vi "Write BBM Slot.vi"(0 "WorkTable Class in":refnum<class "WorkTable Class.lvclass">, 5 "Chuck Number":u32, 7 "Slot Number":u32, 9 "new element/subarray":T1, 11 "error in (no error)":errorcluster) -> (4 "WorkTable Class out":refnum<class "WorkTable Class.lvclass">, 15 "error out":errorcluster)   [LabVIEW 2011, in "WorkTable Class.lvclass"]
uses:
  WorkTable Class.lvclass
  Vec3d Class/Vec3d Class.lvclass
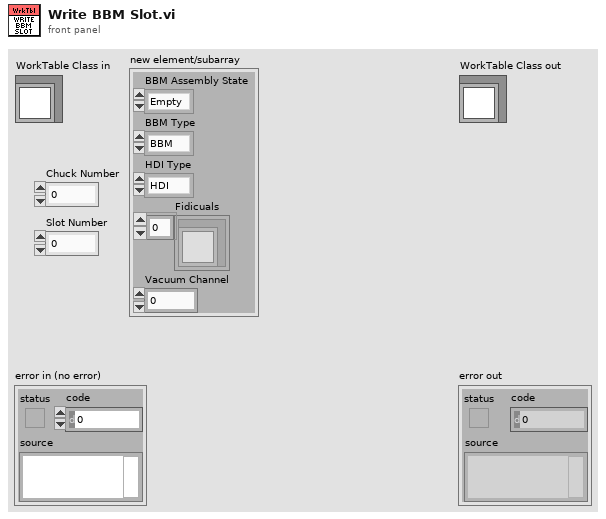
[diagram p1: front panel]
types:
  T1 = cluster{"BBM Assembly State":enum16{"Empty", "Unglued", "Stamped", "PartOnTop", "Weighted"}, "BBM Type":enum16{"BBM", "GlassSlide"}, "HDI Type":enum16{"HDI", "Polyimide"}, "Fidicuals":refnum<class "Vec3d Class.lvclass">[], "Vacuum Channel":u8}
  T2 = cluster{"BBM Chucks":cluster{"BBM Slots":cluster{"BBM Assembly State":enum16{"Empty", "Unglued", "Stamped", "PartOnTop", "Weighted"}, "BBM Type":enum16{"BBM", "GlassSlide"}, "HDI Type":enum16{"HDI", "Polyimide"}, "Fidicuals":refnum<class "Vec3d Class.lvclass">[], "Vacuum Channel":u8}[]}[]}
  T3 = cluster{"BBM Slots":cluster{"BBM Assembly State":enum16{"Empty", "Unglued", "Stamped", "PartOnTop", "Weighted"}, "BBM Type":enum16{"BBM", "GlassSlide"}, "HDI Type":enum16{"HDI", "Polyimide"}, "Fidicuals":refnum<class "Vec3d Class.lvclass">[], "Vacuum Channel":u8}[]}[]
  T4 = cluster{"BBM Slots":cluster{"BBM Assembly State":enum16{"Empty", "Unglued", "Stamped", "PartOnTop", "Weighted"}, "BBM Type":enum16{"BBM", "GlassSlide"}, "HDI Type":enum16{"HDI", "Polyimide"}, "Fidicuals":refnum<class "Vec3d Class.lvclass">[], "Vacuum Channel":u8}[]}
  T5 = cluster{"BBM Assembly State":enum16{"Empty", "Unglued", "Stamped", "PartOnTop", "Weighted"}, "BBM Type":enum16{"BBM", "GlassSlide"}, "HDI Type":enum16{"HDI", "Polyimide"}, "Fidicuals":refnum<class "Vec3d Class.lvclass">[], "Vacuum Channel":u8}[]
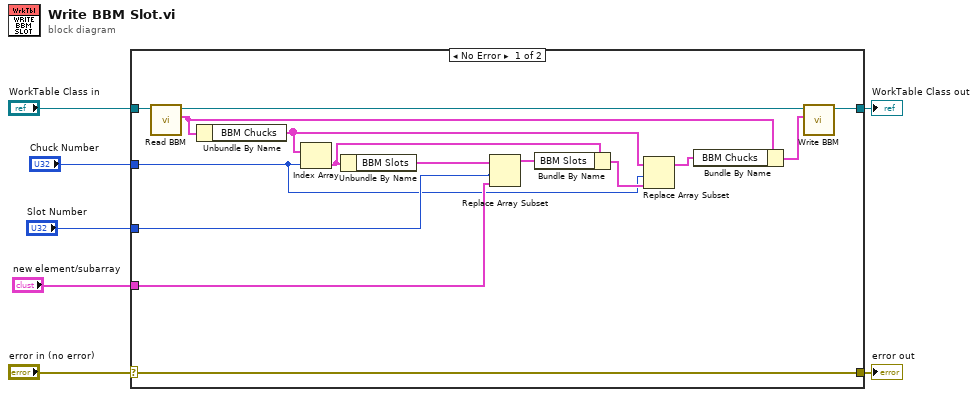
[diagram p0: block diagram]
diagram:
  n1 = case shown="No Error" "error in (no error)" {
    selector: "error in (no error)" -> [w22 w24]
    tunnel: [w22 w24] -> w6
    tunnel: [w9 w23] -> w4
    tunnel: "WorkTable Class in" -> [w21 w23]
    tunnel: "Chuck Number" -> [w13 _]
    tunnel: "Slot Number" -> [w19 _]
    tunnel: "new element/subarray" -> [w18 _]
    frame No Error {
      n2 = call-dynamic "Read BBM.vi"("WorkTable Class in"=w21) -> ("BBM"=w12:T2, "WorkTable Class out"=w10:refnum<class "WorkTable Class.lvclass">)  [unwired: 8 in, 1 out]
      n3 = Unbundle By Name(w12) -> ("BBM Chucks"=w15:T3)
      n4 = Index Array(array=w15, index=w13) -> (element=w17:T4)
      n5 = Unbundle By Name(w17) -> ("BBM Slots"=w20:T5)
      n6 = Replace Array Subset(array=w20, new element=w18, index=w19) -> (w16:T5)
      n7 = Bundle By Name(cluster=w17, "BBM Slots"=w16) -> (w14:T4)
      n8 = Replace Array Subset(array=w15, new element=w14, index=w13) -> (w11:T3)
      n9 = Bundle By Name(cluster=w12, "BBM Chucks"=w11) -> (w8:T2)
      n10 = call-dynamic "Write BBM.vi"("BBM"=w8, "WorkTable Class in"=w10) -> ("WorkTable Class out"=w9:refnum<class "WorkTable Class.lvclass">)  [unwired: 8 in, 1 out]
    }
    frame Error {
    }
  }
  "error out" <- w6
  "WorkTable Class out" <- w4
